vi "R-T Data Input [Spreadsheet].vi"() -> (1 "Kelvin-ohm":cluster{"T [Kelvin]":dbl[], "R [ohm]":dbl[]}, 2 "Celsius -kilohm":cluster{"T [Celsius]":dbl[], "R [kilohm]":dbl[]})   [LabVIEW 2017]
uses:
  <vilib>/Utility/file.llb/Read Delimited Spreadsheet (DBL).vi
panel:
  out "XY Graph":cluster{"all rows":dbl[], "all rows":dbl[]}(graph)
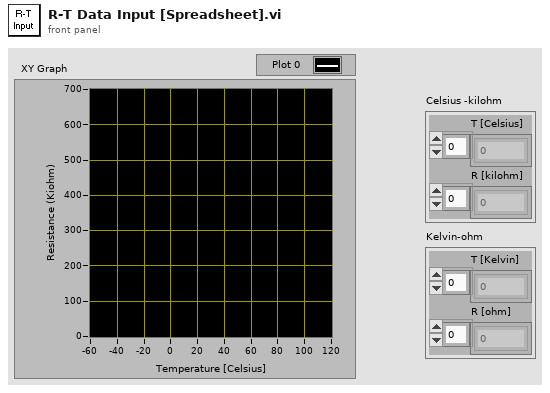
[diagram p1: front panel]
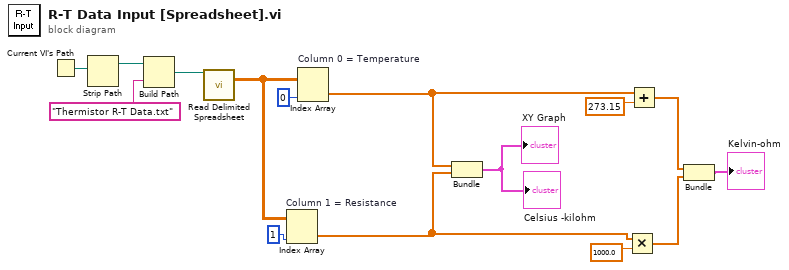
[diagram p0: block diagram]
diagram:
  n1 = Current VI's Path() -> (path=w13:path)
  n2 = Strip Path(path=w13) -> (stripped path=w12:path)  [unwired: 1 out]
  n3 = Build Path(base path=w12, name or relative path="Thermistor R-T Data.txt") -> (appended path=w14:path)
  n4 = call-poly <vilib>:"Read Delimited Spreadsheet.vi"("file path (dialog if empty)"=w14) -> ("all rows"=w9:dbl[][])  [unwired: 9 in, 5 out]
  n5 = Index Array "Column 1 = Resistance"(array=w9, index (col)=1 ("disabled index (col)")) -> (element=w4:dbl[])  [unwired: 1 in]
  n6 = Index Array "Column 0 = Temperature"(array=w9, index (col)=0 ("disabled index (col)")) -> (element=w5:dbl[])  [unwired: 1 in]
  n7 = Bundle("all rows"=w5, "all rows"=w4) -> (→"XY Graph" →"Celsius -kilohm":cluster{"all rows":dbl[], "all rows":dbl[]})  [unwired: 1 in]
  n8 = Multiply(x=w4, y=1000.0) -> (x*y=w2:dbl[])
  n9 = Add(x=w5, y=273.15) -> (x+y=w3:dbl[])
  n10 = Bundle(w3, w2) -> (→"Kelvin-ohm":cluster{dbl[], dbl[]})  [unwired: 1 in]
